vi "Write to Hyperslab.vi"(7 "indices":u64[](array[numeric]), 8 "error in (no error)":errorcluster, 9 "Variant":variant, 10 "Label.Text":string, 11 "Refnum in":T1) -> (0 "error out":errorcluster, 3 "Refnum out":T1)   [LabVIEW 2019, in "HDF5 Tools.lvlib"]
uses:
  <vilib>/UPVI/lvhdf5/library.llb/HDF5 Ref.ctl
  <vilib>/UPVI/lvhdf5/dataset.llb/H5Dwrite (Variant).vi
  <vilib>/UPVI/lvhdf5/dataset.llb/H5Dwrite.xnode
  HDF5 Tools.lvlib
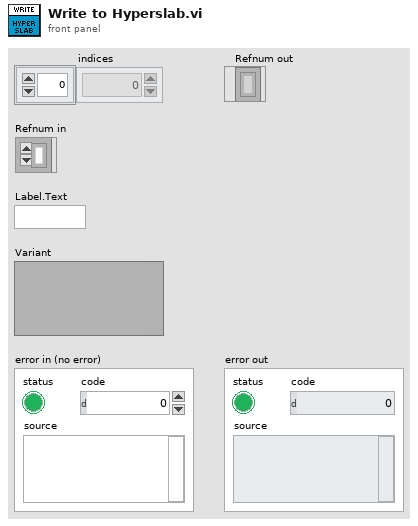
[diagram p1: front panel]
types:
  T1 = typedef "HDF5 Ref.ctl" = refnum<k1>
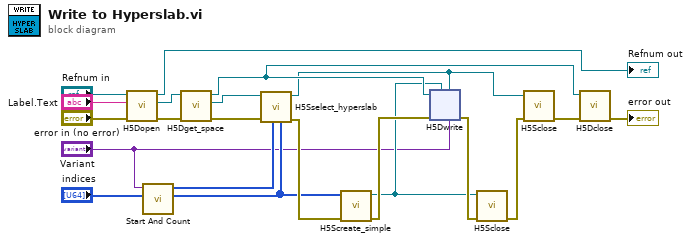
[diagram p0: block diagram]
diagram:
  n1 = call <vilib>:"H5Dopen.vi"("error in (no error)"="error in (no error)", "name"="Label.Text", "HDF5 Ref"="Refnum in") -> ("error out"=w5:errorcluster, "HDF5 Dataset Ref"=w4:T1, "HDF5 Ref out"=→"Refnum out":T1)  [unwired: 4 in]
  n2 = call "Start And Count.vi"("indices"="indices", "Variant"="Variant") -> ("count"=w8:u64[], "start"=w9:u64[])  [unwired: 8 in]
  n3 = call <vilib>:"H5Dget_space.vi"("error in (no error)"=w5, "HDF5 Dataset Ref"=w4) -> ("error out"=w6:errorcluster, "HDF5 Dataspace Ref"=w10:T1, "HDF5 Dataset Ref out"=w18:T1)  [unwired: 5 in]
  n4 = call <vilib>:"H5Sselect_hyperslab.vi"("Count"=w8, "Start"=w9, "error in (no error)"=w6, "HDF5 Space Ref"=w10) -> ("error out"=w19:errorcluster, "HDF5 Ref out"=w13:T1)  [unwired: 6 in]
  n5 = call <vilib>:"H5Screate_simple.vi"("error in (no error)"=w19, "Dimensions"=w8) -> ("error out"=w20:errorcluster, "HDF5 Ref out"=w12:T1)  [unwired: 6 in]
  n6 = xnode "H5Dwrite"("HDF5 Dataset Ref"=w18, "HDF5 File Space Ref (H5S_ALL)"=w13, "HDF5 Memory Space Ref (H5S_ALL)"=w12, "error in (no error)"=w20, "Data"="Variant") -> ("error out"=w14:errorcluster)  [unwired: 2 in, 1 out]
  n7 = call <vilib>:"H5Sclose.vi"("error in (no error)"=w14, "HDF5 Dataspace Ref"=w12) -> ("error out"=w15:errorcluster)  [unwired: 7 in]
  n8 = call <vilib>:"H5Sclose.vi"("error in (no error)"=w15, "HDF5 Dataspace Ref"=w13) -> ("error out"=w16:errorcluster)  [unwired: 7 in]
  n9 = call <vilib>:"H5Dclose.vi"("error in (no error)"=w16, "HDF5 Dataset Ref"=w18) -> ("error out"=→"error out":errorcluster)  [unwired: 7 in]
